vi "Dispensing on baseplate.vi"   [LabVIEW 2016]
uses:
  Classes/Workspace/Carrier Tray/Syringe Space/Syringe Space.lvclass
  Classes/Workspace/Carrier Tray/Assembly Tray.lvclass
  Classes/Routine/Secure Syringe/SecureRelease Syringe.lvclass
  Classes/Routine/Dispense/Iterative Dispense/8 inch/8 inch Baseplate Dispense.lvclass
  Classes/Routine/Dispense/CAD Dispense/8 inch Sensor Dispense.lvclass
  Classes/Routine/Secure Syringe/SecureRelease Syringe.lvclass/SecureRelease Syringe.ctl
  Classes/Routine/Secure Syringe/Write Type.vi
  Classes/Controller/Controller.lvclass
types:
  T1 = typedef "Controller.lvclass/Controllers.ctl" = cluster{"I-O.lvclass":refnum<class "I-O.lvclass">, "Motion.lvclass":refnum<class "Motion.lvclass">, "Dispenser.lvclass":refnum<class "Dispenser.lvclass">}
  T2 = typedef "Fixture.lvclass/Workspace.ctl" = cluster{"XYZTheta":dbl[], "Workspace Valve":i32, "Workspace Sensor":i32}
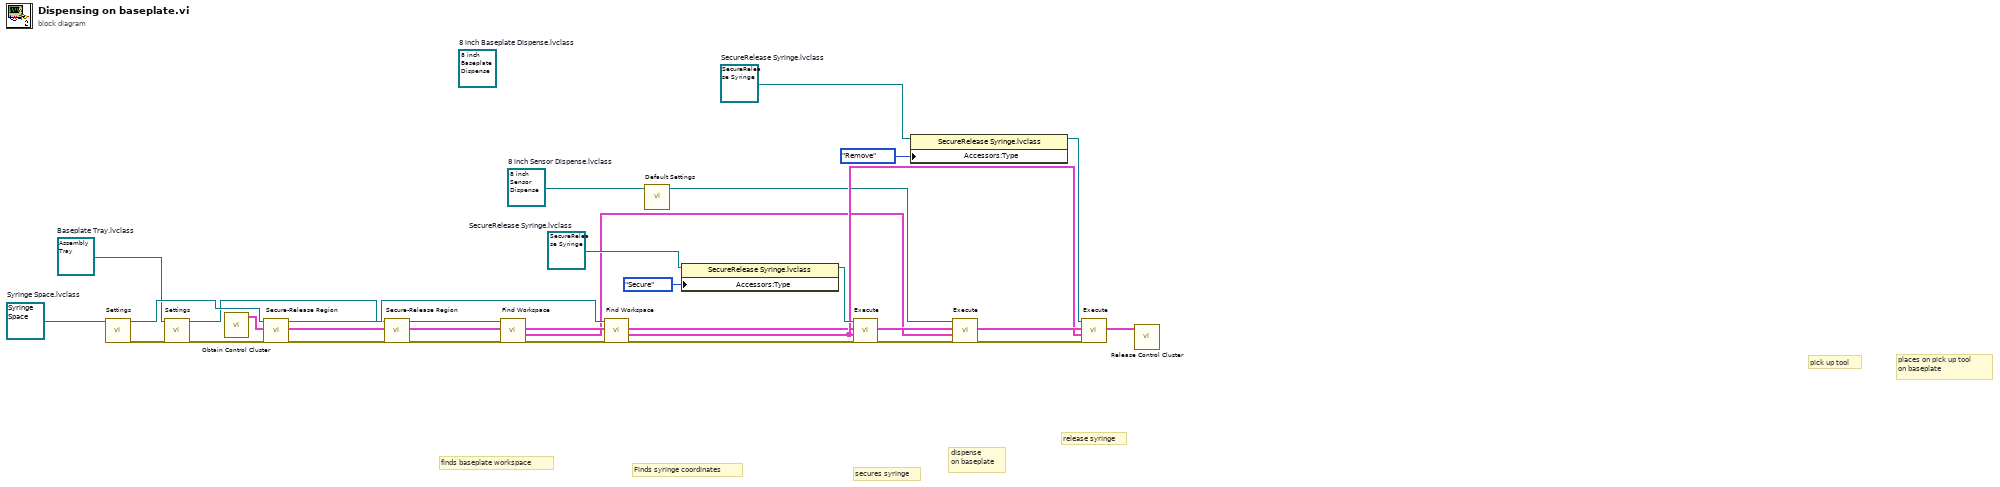
[diagram p0: block diagram]
diagram:
  w2 = refnum<class "8 inch Sensor Dispense.lvclass"> refnum  # 8 inch Sensor Dispense.lvclass
  (unwired) refnum<class "8 inch Baseplate Dispense.lvclass"> refnum  # 8 inch Baseplate Dispense.lvclass
  w17 = refnum<class "SecureRelease Syringe.lvclass"> refnum  # SecureRelease Syringe.lvclass
  w26 = refnum<class "Assembly Tray.lvclass"> refnum  # Baseplate Tray.lvclass
  w29 = refnum<class "SecureRelease Syringe.lvclass"> refnum  # SecureRelease Syringe.lvclass
  w32 = refnum<class "Syringe Space.lvclass"> refnum  # Syringe Space.lvclass
  # "places on pick up tool\non baseplate"
  # "pick up tool"
  # "release syringe"
  # "dispense\non baseplate"
  # "secures syringe"
  # "Finds syringe coordinates"
  # "finds baseplate workspace"
  n1 = call-dynamic "Settings.vi"("Syringe Space in"=w32) -> ("error out"=w18:errorcluster, "Syringe Space out"=w31:refnum<class "Syringe Space.lvclass">)  [unwired: 9 in]
  n2 = call-dynamic "Settings.vi"("error in (no error)"=w18, "Baseplate Tray In"=w26) -> ("error out"=w5:errorcluster, "Baseplate Tray Out"=w23:refnum<class "Assembly Tray.lvclass">)  [unwired: 8 in]
  n3 = call "Obtain Control Cluster.vi"() -> ("Control Out"=w22:T1)  [unwired: 11 in]
  n4 = call-dynamic "Secure-Release Region.vi"("error in (no error)"=w5, "Control In"=w22, "Baseplate Tray in"=w31) -> ("error out"=w11:errorcluster, "Control Out"=w21:T1, "Baseplate Tray out"=w30:refnum<class "Syringe Space.lvclass">)  [unwired: 6 in]
  n5 = call-dynamic "Secure-Release Region.vi"("error in (no error)"=w11, "Control In"=w21, "Baseplate Tray in"=w23) -> ("error out"=w10:errorcluster, "Control Out"=w25:T1, "Baseplate Tray out"=w24:refnum<class "Assembly Tray.lvclass">)  [unwired: 6 in]
  n6 = call-dynamic "Find Workspace.vi"("Error In"=w10, "Control In"=w25, "Baseplate Tray in"=w24) -> ("Error Out"=w9:errorcluster, "Workspace"=w12:T2, "Control Out"=w20:T1)  [unwired: 5 in, 1 out]
  n7 = call-dynamic "Find Workspace.vi"("Error In"=w9, "Control In"=w20, "Baseplate Tray in"=w30) -> ("Error Out"=w3:errorcluster, "Workspace"=w13:T2, "Control Out"=w4:T1)  [unwired: 5 in, 1 out]
  n8 = call-dynamic "Default Settings.vi"("8 Inch CAD Dispense in"=w2) -> ("8 Inch CAD Dispense out"=w1:refnum<class "8 inch Sensor Dispense.lvclass">)  [unwired: 9 in, 1 out]
  n9 = property class="SecureRelease Syringe.lvclass"(reference=w29, "Accessors:Type"=enum16{"Secure", "Remove"}."Secure" ("Type")) -> (reference out=w27:refnum<class "SecureRelease Syringe.lvclass">)  [unwired: 1 in, 1 out]
  n10 = call-dynamic "Execute.vi"("error in (no error)"=w3, "Workspace"=w13, "Control In"=w4, "Secure Syringe in"=w27) -> ("error out"=w8:errorcluster, "Control Out"=w19:T1)  [unwired: 5 in, 1 out]
  n11 = property class="SecureRelease Syringe.lvclass"(reference=w17, "Accessors:Type"=enum16{"Secure", "Remove"}."Remove" ("Type")) -> (reference out=w15:refnum<class "SecureRelease Syringe.lvclass">)  [unwired: 1 in, 1 out]
  n12 = call-dynamic "Execute.vi"("Error In"=w8, "Workspace"=w12, "Control In"=w19, "Dispense in"=w1) -> ("Error Out"=w7:errorcluster, "Control Out"=w14:T1)  [unwired: 5 in, 1 out]
  n13 = call-dynamic "Execute.vi"("error in (no error)"=w7, "Workspace"=w13, "Control In"=w14, "Secure Syringe in"=w15) -> ("Control Out"=w6:T1)  [unwired: 5 in, 2 out]
  n14 = call "Release Control Cluster.vi"("output cluster"=w6) -> ()  [unwired: 11 in]
